vi "Configure PID.vi"(0 "VISA resource name":refnum<visa-resource-name>, 5 "Motor ID (0)":u8, 7 "PID Parameters":T1={"Kd (0)"=0.0, "Ki (0)"=0.0, "Kp (4)"=4.0}, 11 "error in (no error)":errorcluster) -> (4 "VISA resource name out":refnum<visa-resource-name>, 15 "error out":errorcluster)   [LabVIEW 2016, in "Dynamixel Motor.lvlib"]
doc: "Sets PID parameters for the motor."
uses:
  Dynamixel Motor.lvlib
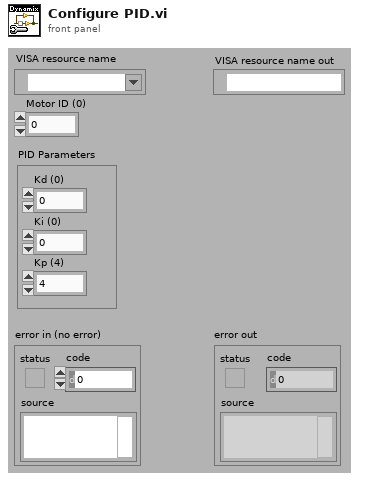
[diagram p1: front panel]
types:
  T1 = cluster{"Kd (0)":dbl, "Ki (0)":dbl, "Kp (4)":dbl}
  T2 = enum16{"big-endian, network order", "native, host order", "little-endian"}
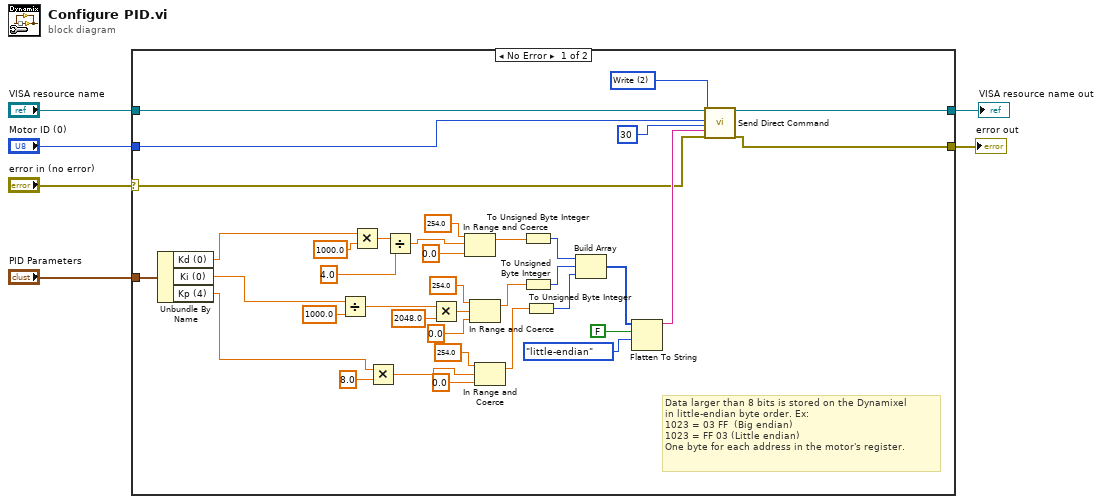
[diagram p0: block diagram]
diagram:
  n1 = case shown="No Error" "error in (no error)" {
    selector: "error in (no error)" -> [w27 w45]
    tunnel: "VISA resource name" -> [w43 w44]
    tunnel: [w42 w44] -> w5
    tunnel: [w41 w45] -> w4
    tunnel: "Motor ID (0)" -> [w40 _]
    tunnel: "PID Parameters" -> [w10 _]
    frame No Error {
      w12 = u16 2 items=["Ping", "Read", "Write", "Registered Write", "Action", "Reset", "Sync Write"] ("Select Action")
      # "Data larger than 8 bits is stored on the Dynamixel \nin little-endian byte order. Ex:\n1023 = 03 FF  (Big endian)\n1023 = FF 03 (Little endian)\nOne byte for each address in the motor's register."
      n2 = Unbundle By Name(w10) -> ("Kd (0)"=w9:dbl, "Ki (0)"=w8:dbl, "Kp (4)"=w7:dbl)
      n3 = Divide(x=w8, y=1000.0 ("Maximum RPM")) -> (x/y=w35:dbl)
      n4 = Multiply(x=w9, y=1000.0) -> (x*y=w16:dbl)
      n5 = Multiply(x=w7, y=8.0) -> (x*y=w17:dbl)
      n6 = Divide(x=w16, y=4.0) -> (x/y=w15:dbl)
      n7 = Multiply(x=w35, y=2048.0 ("upper limit")) -> (x*y=w38:dbl)
      n8 = In Range and Coerce(upper limit=254.0, x=w15, lower limit=0.0) -> (coerced(x)=w24:dbl)  [unwired: 1 out]
      n9 = In Range and Coerce(upper limit=254.0, x=w38, lower limit=0.0) -> (coerced(x)=w29:dbl)  [unwired: 1 out]
      n10 = In Range and Coerce(upper limit=254.0, x=w17, lower limit=0.0) -> (coerced(x)=w19:dbl)  [unwired: 1 out]
      n11 = To Unsigned Byte Integer(number=w24) -> (unsigned 8bit integer=w30:u8)
      n12 = To Unsigned Byte Integer(number=w29) -> (unsigned 8bit integer=w21:u8)
      n13 = To Unsigned Byte Integer(number=w19) -> (unsigned 8bit integer=w20:u8)
      n14 = Build Array(w30, w21, w20) -> (w13:u8[])
      n15 = Flatten To String(anything=w13, prepend array or string size? (T)=FALSE, byte order (0:big-endian, network order)=T2."little-endian") -> (data string=w28:string)  [unwired: 1 in, 2 out]
      n16 = call "Send Direct Command.vi"("VISA resource name"=w43, "Select Action"=w12, "Motor ID (0)"=w40, "Address"=u8 30, "Parameters"=w28, "Error in (no error)"=w27) -> ("VISA resource name out"=w42:refnum<visa-resource-name>, "Error out"=w41:errorcluster)  [unwired: 11 in, 1 out]
    }
    frame Error {
    }
  }
  "VISA resource name out" <- w5
  "error out" <- w4
